vi "picoquant_check_loop_notifier.vi"(8 "error in (no error)":errorcluster, 11 "picoquant_generic in":refnum<class "picoquant_generic.lvclass">) -> (0 "error out":errorcluster, 2 "exit?":bool, 3 "picoquant_generic out":refnum<class "picoquant_generic.lvclass">)   [LabVIEW 2015, in "picoquant_generic.lvclass"]
uses:
  picoquant_generic.lvclass
  picoquant_generic.lvclass/picoquant_generic.ctl
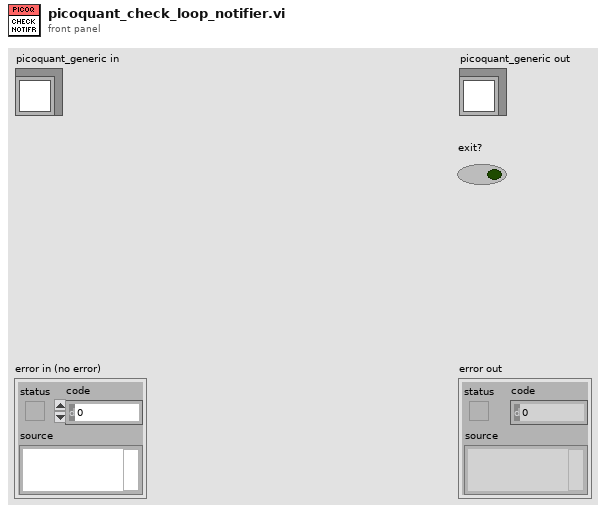
[diagram p1: front panel]
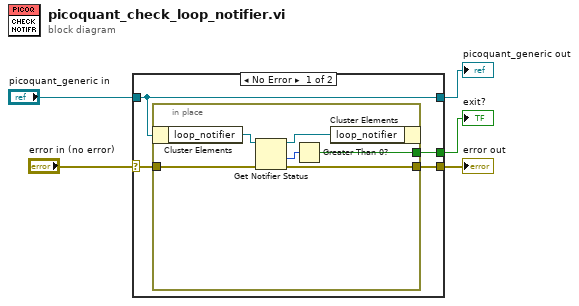
[diagram p0: block diagram]
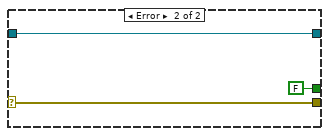
[diagram p2: hidden frame]
diagram:
  n1 = case shown="No Error" "error in (no error)" {
    selector: "error in (no error)" -> [w8 w18]
    tunnel: [w7 w18] -> w4
    tunnel: [w9 w17] -> w2
    tunnel: "picoquant_generic in" -> [w9 w17]
    tunnel: [w6 FALSE] -> w1
    frame No Error {
      n2 = in-place {
        in-place-border: w8 -> [w14]
        in-place-border: [w13] -> w7
        in-place-border: [w10] -> w6
        n3 = in-place-cluster #1(w9) -> ("loop_notifier"=w15:refnum<notifier>)
        n4 = Get Notifier Status(notifier=w15, error in (no error)=w14) -> (notifier out=w12:refnum<notifier>, # waiting=w11:i32, error out=w13:errorcluster)  [unwired: 2 out]
        n5 = Greater Than 0?(x=w11) -> (x > 0?=w10:bool)
        n6 = in-place-cluster #1("loop_notifier"=w12) -> ()  [unwired: 1 out]
      }
    }
    frame Error {
    }
  }
  "error out" <- w4
  "picoquant_generic out" <- w2
  "exit?" <- w1
